vi "Pre Launch Init.vi"(11 "Nested in":refnum<class "UI.lvclass">) -> (0 "error out":errorcluster, 3 "Nested out":refnum<class "UI.lvclass">)   [LabVIEW 2020, in "UI.lvlib" / "UI.lvclass"]
doc: "(<B>Filename</B>: Actor Framework.lvlib:Actor.lvclass:Pre Launch Init.vi)\n\nDefines behavior that occurs after the Launch Nested Actor method is invoked but before the actor's Actor Core method begins running.\n\nBy default, this method does nothing. A descendant class may override it to define behavior."
uses:
  UI.lvclass
  <vilib>/ActorFramework/Actor/Actor.lvclass
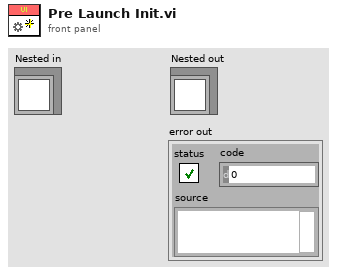
[diagram p1: front panel]
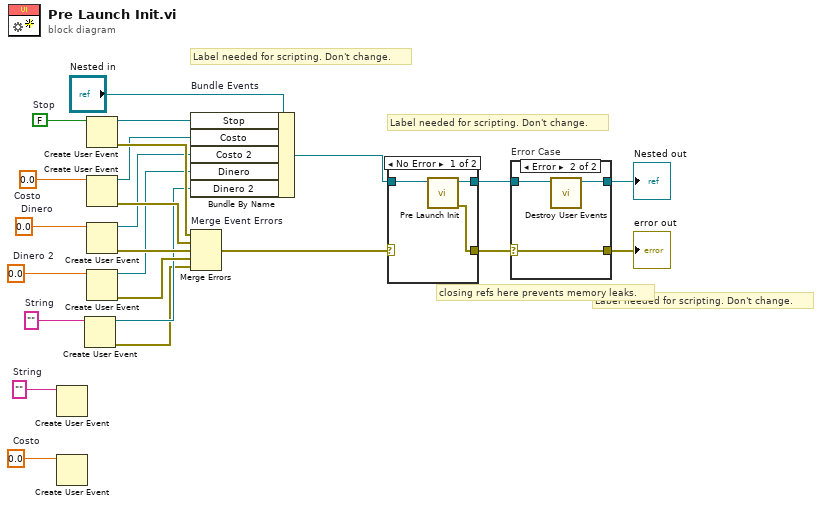
[diagram p0: block diagram]
diagram:
  w3 = ""  # String
  w4 = ""  # String
  w7 = 0.0  # Dinero 2
  w10 = 0.0  # Dinero
  w13 = 0.0  # Costo
  w14 = 0.0  # Costo
  w23 = FALSE  # Stop
  # "Label needed for scripting. Don't change."
  # "Label needed for scripting. Don't change."
  # "Label needed for scripting. Don't change."
  # "closing refs here prevents memory leaks."
  n1 = Create User Event(user event datatype=w4) -> ()  [unwired: 1 in, 2 out]
  n2 = Create User Event(user event datatype=w14) -> ()  [unwired: 1 in, 2 out]
  n3 = Create User Event(user event datatype=w3) -> (user event=w2:refnum<user-event>, error out=w1:errorcluster)  [unwired: 1 in]
  n4 = Create User Event(user event datatype=w23) -> (user event=w20:refnum<user-event>, error out=w22:errorcluster)  [unwired: 1 in]
  n5 = Create User Event(user event datatype=w13) -> (user event=w12:refnum<user-event>, error out=w11:errorcluster)  [unwired: 1 in]
  n6 = Create User Event(user event datatype=w10) -> (user event=w9:refnum<user-event>, error out=w8:errorcluster)  [unwired: 1 in]
  n7 = Create User Event(user event datatype=w7) -> (user event=w6:refnum<user-event>, error out=w5:errorcluster)  [unwired: 1 in]
  n8 = Bundle By Name "Bundle Events"(cluster="Nested in", "Stop"=w20, "Costo"=w12, "Costo 2"=w9, "Dinero"=w6, "Dinero 2"=w2) -> (w17:refnum<class "UI.lvclass">)
  n9 = Merge Errors "Merge Event Errors"(w22, w11, w8, w5, w1) -> (w16:errorcluster)
  n10 = case shown="No Error" w16 {
    selector: w16 -> [_ w29]
    tunnel: [w27 w28] -> w18
    tunnel: w17 -> [w26 w28]
    tunnel: [w25 w29] -> w15
    frame No Error {
      n11 = call-parent "Pre Launch Init.vi"("Actor in"=w26) -> ("error out"=w25:errorcluster, "Actor out"=w27:refnum<class "UI.lvclass">)  [unwired: 9 in]
    }
    frame Error {
    }
  }
  n12 = case "Error Case" shown="Error" w15 {
    selector: w15 -> [w30 w34]
    tunnel: w18 -> [w31 w33]
    tunnel: [w31 w32] -> w21
    tunnel: [w30 w34] -> w19
    frame No Error {
    }
    frame Error {
      n13 = call "Destroy User Events.vi"("UI Template in"=w33) -> ("UI Template out"=w32:refnum<class "UI.lvclass">)  [unwired: 10 in]
    }
  }
  "error out" <- w19
  "Nested out" <- w21
